vi "Delta_P_inc_neg.vi"() -> (5 "Plug in titles":string[](array[string]), 7 "Plug in values":string[](array[string]))   [LabVIEW 2010]
uses:
  Globals/Plug_in_data_global.vi
  Globals/Meas_global.vi
panel:
  out "D,D/2":dbl[](graph)
  out "Flange":dbl[](graph)
  out "Corner":dbl[](graph)
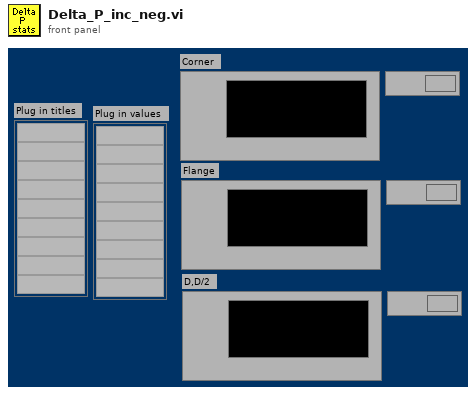
[diagram p1: front panel]
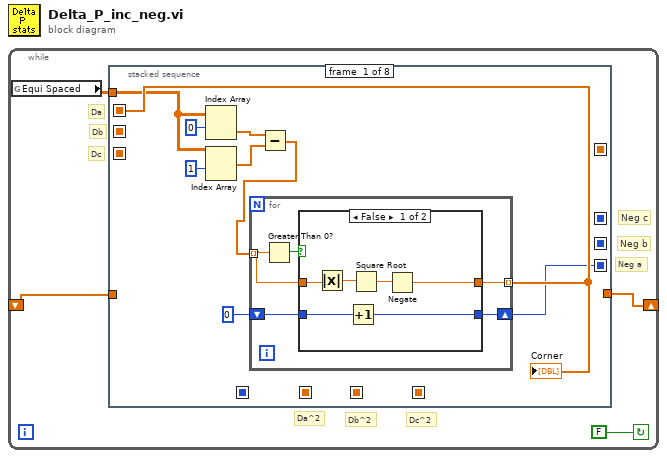
[diagram p0: block diagram]
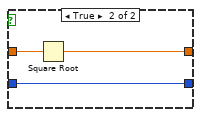
[diagram p2: hidden frame]
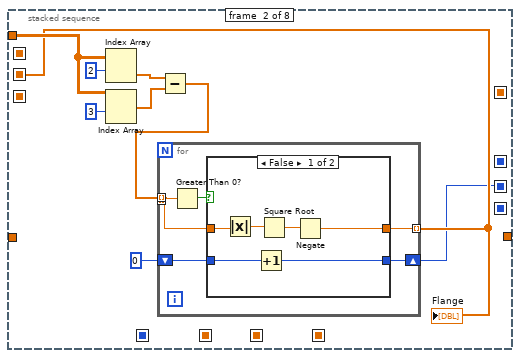
[diagram p3: hidden frame]
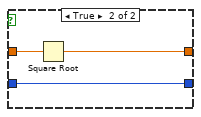
[diagram p4: hidden frame]
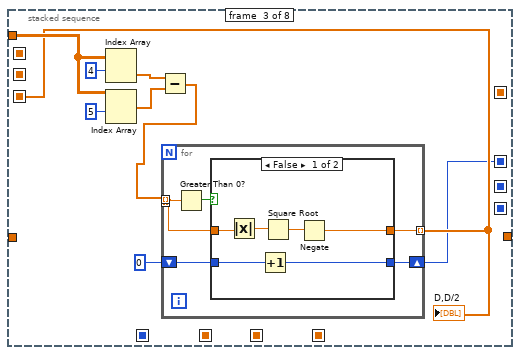
[diagram p5: hidden frame]
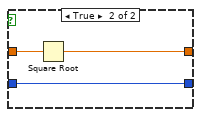
[diagram p6: hidden frame]
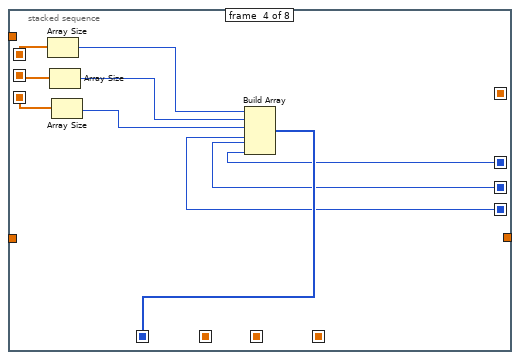
[diagram p7: hidden frame]
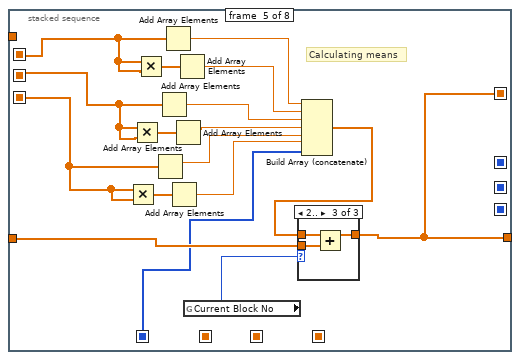
[diagram p8: hidden frame]
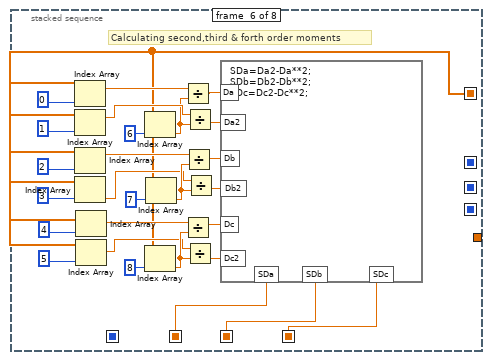
[diagram p11: hidden frame]
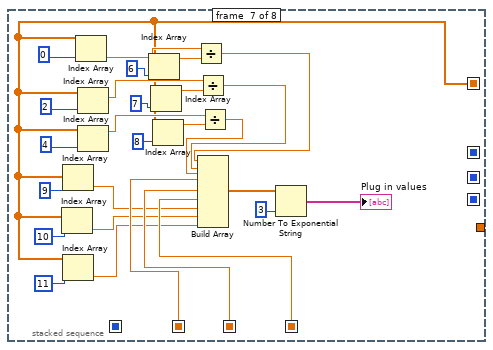
[diagram p12: hidden frame]
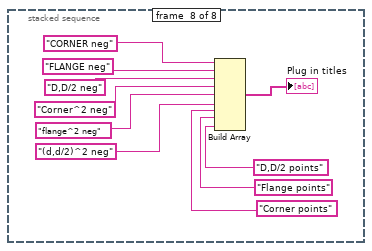
[diagram p13: hidden frame]
diagram:
  n1 = while {
    shift-left: _ -> [w4]
    shift-right: [w3] -> _
    stop <- FALSE continue-if-true
    # "Neg c"
    # "Neg b"
    # "Neg a"
    # "Dc^2"
    # "Db^2"
    # "Da^2"
    # "Dc"
    # "Db"
    # "Da"
    n2 = global read "Plug_in_data_global.vi" "Equi Spaced"() -> (w2:dbl[][])
    n3 = stacked-sequence {
      seq-local: [_ _ _ _ _ w126 _ _] -> [_ _ _ _ _ _ w160 _]
      seq-local: [_ _ _ _ w88 _ _ _] -> [_ _ _ _ _ w110 w140 _]
      seq-local: [_ _ _ _ _ w127 _ _] -> [_ _ _ _ _ _ w161 _]
      seq-local: [_ _ _ _ _ w125 _ _] -> [_ _ _ _ _ _ w157 _]
      seq-local: [w8 _ _ _ _ _ _ _] -> [_ _ _ w79 w90 _ _ _]
      seq-local: [_ w30 _ _ _ _ _ _] -> [_ _ _ w78 w89 _ _ _]
      seq-local: [_ _ w53 _ _ _ _ _] -> [_ _ _ w77 w84 _ _ _]
      seq-local: [w5 _ _ _ _ _ _ _] -> [_ _ _ w74 _ _ _ _]
      seq-local: [_ w28 _ _ _ _ _ _] -> [_ _ _ w75 _ _ _ _]
      seq-local: [_ _ w51 _ _ _ _ _] -> [_ _ _ w76 _ _ _ _]
      seq-local: [_ _ _ w83 _ _ _ _] -> [_ _ _ _ w85 _ _ _]
      tunnel: w4 -> [_ _ _ _ w98 _ _ _]
      tunnel: [_ _ _ _ w88 _ _ _] -> w3
      tunnel: w2 -> [w7 w32 w55 _ _ _ _ _]
      frame #0 {
        n4 = Index Array(array=w7, index (row)=0) -> (element=w11:dbl[])  [unwired: 1 in]
        n5 = Index Array(array=w7, index (row)=1) -> (element=w10:dbl[])  [unwired: 1 in]
        n6 = Subtract(x=w11, y=w10) -> (x-y=w9:dbl[])
        n7 = for {
          tunnel: w9 -> [w17] mode=indexing
          tunnel: [w16] -> w8 mode=indexing
          shift-right: [w14] -> w5
          shift-left: 0 -> [w15]
          n8 = Greater Than 0?(x=w17) -> (x > 0?=w18:bool)
          n9 = case shown="False" w18 {
            tunnel: w17 -> [w24 w26]
            tunnel: [w21 w27] -> w16
            tunnel: w15 -> [w20 w25]
            tunnel: [w19 w25] -> w14
            frame False {
              n10 = Absolute Value(x=w24) -> (abs(x)=w23:dbl)
              n11 = Increment(x=w20) -> (x+1=w19:i32)
              n12 = Square Root(x=w23) -> (sqrt(x)=w22:dbl)
              n13 = Negate(x=w22) -> (-x=w21:dbl)
            }
            frame True {
              n14 = Square Root(x=w26) -> (sqrt(x)=w27:dbl)
            }
          }
        }
        "Corner" <- w8
      }
      frame #1 {
        n15 = Index Array(array=w32, index (row)=2) -> (element=w34:dbl[])  [unwired: 1 in]
        n16 = Index Array(array=w32, index (row)=3) -> (element=w33:dbl[])  [unwired: 1 in]
        n17 = Subtract(x=w34, y=w33) -> (x-y=w31:dbl[])
        n18 = for {
          tunnel: [w37] -> _ mode=indexing
          tunnel: [w40] -> w30 mode=indexing
          shift-right: [w38] -> w28
          shift-left: 0 -> [w39]
          tunnel: w31 -> [w37] mode=indexing
          n19 = Greater Than 0?(x=w37) -> (x > 0?=w41:bool)
          n20 = case shown="False" w41 {
            tunnel: w37 -> [w47 w49]
            tunnel: [w44 w50] -> w40
            tunnel: w39 -> [w43 w48]
            tunnel: [w42 w48] -> w38
            frame False {
              n21 = Absolute Value(x=w47) -> (abs(x)=w46:dbl)
              n22 = Increment(x=w43) -> (x+1=w42:i32)
              n23 = Square Root(x=w46) -> (sqrt(x)=w45:dbl)
              n24 = Negate(x=w45) -> (-x=w44:dbl)
            }
            frame True {
              n25 = Square Root(x=w49) -> (sqrt(x)=w50:dbl)
            }
          }
        }
        "Flange" <- w30
      }
      frame #2 {
        n26 = Index Array(array=w55, index (row)=4) -> (element=w57:dbl[])  [unwired: 1 in]
        n27 = Index Array(array=w55, index (row)=5) -> (element=w56:dbl[])  [unwired: 1 in]
        n28 = Subtract(x=w57, y=w56) -> (x-y=w54:dbl[])
        n29 = for {
          tunnel: [w60] -> _ mode=indexing
          tunnel: [w63] -> w53 mode=indexing
          shift-right: [w61] -> w51
          shift-left: 0 -> [w62]
          tunnel: w54 -> [w60] mode=indexing
          n30 = Greater Than 0?(x=w60) -> (x > 0?=w64:bool)
          n31 = case shown="False" w64 {
            tunnel: w60 -> [w70 w72]
            tunnel: [w67 w73] -> w63
            tunnel: w62 -> [w66 w71]
            tunnel: [w65 w71] -> w61
            frame False {
              n32 = Absolute Value(x=w70) -> (abs(x)=w69:dbl)
              n33 = Increment(x=w66) -> (x+1=w65:i32)
              n34 = Square Root(x=w69) -> (sqrt(x)=w68:dbl)
              n35 = Negate(x=w68) -> (-x=w67:dbl)
            }
            frame True {
              n36 = Square Root(x=w72) -> (sqrt(x)=w73:dbl)
            }
          }
        }
        "D,D/2" <- w53
      }
      frame #3 {
        n37 = Array Size(array=w79) -> (size(s)=w82:i32)
        n38 = Array Size(array=w78) -> (size(s)=w81:i32)
        n39 = Array Size(array=w77) -> (size(s)=w80:i32)
        n40 = Build Array(w82, w81, w80, w74, w75, w76) -> (w83:i32[])
      }
      frame #4 {
        # "Calculating means"
        n41 = Multiply(x=w84, y=w84) -> (x*y=w95:dbl[])
        n42 = Multiply(x=w89, y=w89) -> (x*y=w96:dbl[])
        n43 = Multiply(x=w90, y=w90) -> (x*y=w97:dbl[])
        n44 = Add Array Elements(numeric array=w84) -> (sum=w92:dbl)
        n45 = Add Array Elements(numeric array=w89) -> (sum=w94:dbl)
        n46 = Add Array Elements(numeric array=w90) -> (sum=w100:dbl)
        n47 = Add Array Elements(numeric array=w95) -> (sum=w91:dbl)
        n48 = Add Array Elements(numeric array=w96) -> (sum=w93:dbl)
        n49 = Add Array Elements(numeric array=w97) -> (sum=w99:dbl)
        n50 = global read "Meas_global.vi" "Current Block No"() -> (w87:i32)
        n51 = Build Array (concatenate)(w100, w99, w94, w93, w92, w91, w85) -> (w86:dbl[])
        n52 = case shown="2.." w87 {
          tunnel: [w101 w102 w105] -> w88
          tunnel: w98 -> [_ _ w104]
          tunnel: w86 -> [w101 w102 w103]
          frame ..0 {
          }
          frame 1 {
          }
          frame 2.. {
            n53 = Add(x=w103, y=w104) -> (x+y=w105:dbl[])
          }
        }
      }
      frame #5 {
        # "Calculating second,third & forth order moments"
        n54 = Index Array(array=w110, index=0) -> (element=w122:dbl)
        n55 = Index Array(array=w110, index=1) -> (element=w123:dbl)
        n56 = Index Array(array=w110, index=2) -> (element=w114:dbl)
        n57 = Index Array(array=w110, index=3) -> (element=w113:dbl)
        n58 = Index Array(array=w110, index=4) -> (element=w112:dbl)
        n59 = Index Array(array=w110, index=5) -> (element=w111:dbl)
        n60 = Index Array(array=w110, index=6) -> (element=w121:dbl)
        n61 = Index Array(array=w110, index=8) -> (element=w115:dbl)
        n62 = Index Array(array=w110, index=7) -> (element=w118:dbl)
        n63 = Divide(x=w122, y=w121) -> (x/y=w120:dbl)
        n64 = Divide(x=w112, y=w115) -> (x/y=w108:dbl)
        n65 = Divide(x=w114, y=w118) -> (x/y=w106:dbl)
        n66 = Divide(x=w123, y=w121) -> (x/y=w119:dbl)
        n67 = Divide(x=w111, y=w115) -> (x/y=w109:dbl)
        n68 = Divide(x=w113, y=w118) -> (x/y=w107:dbl)
        n69 = formula code="SDa=Da2-Da**2;\nSDb=Db2-Db**2;\nSDc=Dc2-Dc**2;"("Da2"=w119, "Da"=w120, "Db"=w106, "Db2"=w107, "Dc"=w108, "Dc2"=w109) -> ("SDa"=w127:dbl, "SDb"=w126:dbl, "SDc"=w125:dbl)
      }
      frame #6 {
        n70 = Index Array(array=w140, index=10) -> (element=w135:dbl)
        n71 = Index Array(array=w140, index=9) -> (element=w136:dbl)
        n72 = Index Array(array=w140, index=11) -> (element=w134:dbl)
        n73 = Index Array(array=w140, index=0) -> (element=w150:dbl)
        n74 = Index Array(array=w140, index=2) -> (element=w143:dbl)
        n75 = Index Array(array=w140, index=4) -> (element=w144:dbl)
        n76 = Index Array(array=w140, index=6) -> (element=w151:dbl)
        n77 = Index Array(array=w140, index=7) -> (element=w148:dbl)
        n78 = Index Array(array=w140, index=8) -> (element=w145:dbl)
        n79 = Divide(x=w150, y=w151) -> (x/y=w149:dbl)
        n80 = Divide(x=w143, y=w148) -> (x/y=w142:dbl)
        n81 = Divide(x=w144, y=w145) -> (x/y=w141:dbl)
        n82 = Build Array(w149, w142, w141, w161, w160, w157, w136, w135, w134) -> (w158:dbl[])
        n83 = Number To Exponential String(number=w158, precision (6)=3) -> (E-format string=→"Plug in values":string[])  [unwired: 2 in]
      }
      frame #7 {
        n84 = Build Array("CORNER neg", "FLANGE neg", "D,D/2 neg", "Corner^2 neg", "flange^2 neg", "(d,d/2)^2 neg", "Corner points", "Flange points", "D,D/2 points") -> (→"Plug in titles":string[])
      }
    }
  }
